vi "Test Suite Result Fail Count.vi"(8 "error in (no error)":errorcluster, 11 "Test Suite Result Test In":refnum<class "Test Suite Result Test.lvclass">) -> (0 "error out":errorcluster, 3 "Test Suite Result Test Out":refnum<class "Test Suite Result Test.lvclass">)   [LabVIEW 2020, in "LUnit Tests.lvlib" / "Test Suite Result Test.lvclass"]
uses:
  Test Suite Result Test.lvclass
  C:/Program Files (x86)/National Instruments/LabVIEW 2020/vi.lib/Asteme/LUnit/Test Case.lvclass
  source/Examples/Basic Example/Failing Test Case/Failing Test Case.lvclass
  C:/Users/anton/Documents/GitHub/LUnit/source/Framework/Test Case/LUnit Test Case.lvclass
  source/Framework/Result Classes/Test Suite Result/Test Suite Result.lvclass/Test Suite Result.ctl
  source/Framework/Result Classes/Test Case Result/Test Case Result.lvclass/Test Case Result.ctl
  source/Framework/Result Classes/Method Result/Method Result.lvclass/Method Result.ctl
  <vilib>/Asteme/LUnit/Test Case.lvclass/Test Case.ctl
  <vilib>/Asteme/LUnit/LUnit Assertion Result.lvclass/LUnit Assertion Result.ctl
  <vilib>/Asteme/LUnit/LUnit Test Case Result.lvclass/LUnit Test Case Result.ctl
  <vilib>/Asteme/LUnit/LUnit Method Result.lvclass/LUnit Method Result.ctl
  source/Framework/Result Classes/Test Suite Result/Private/SubVIs/Count by Status.vi
  <vilib>/Asteme/LUnit/Palette/Pass.vi
  <vilib>/Asteme/LUnit/Palette/Fail.vi
  <vilib>/Asteme/LUnit/Variant to string.vi
  <vilib>/Asteme/LUnit/Set Assertion Type.vi
  source/Framework/Result Classes/Test Case Result/Public/Accessors/Read Status.vi
  <vilib>/Asteme/LUnit/Add test result.vi
  <vilib>/Asteme/LUnit/LUnit Write Passed.vi
  <vilib>/Asteme/LUnit/LUnit Write Message.vi
  <vilib>/Asteme/LUnit/LUnit Write Description.vi
  <vilib>/Asteme/LUnit/LUnit Write Assertion Type.vi
  source/Framework/Result Classes/Test Case Result/Private/SubVIs/Merge Status.vi
  source/Framework/Result Classes/Method Result/Public/Read Status.vi
  <vilib>/Asteme/LUnit/LUnit Record Assertion Result.vi
  <vilib>/Asteme/LUnit/LUnit Aggregate Assertion Results.vi
  <vilib>/Asteme/LUnit/Assertion Result/LUnit Read Status.vi
  <vilib>/Asteme/LUnit/LUnit Read Message.vi
  <vilib>/Asteme/LUnit/LUnit Read Description.vi
  <vilib>/Asteme/LUnit/Method Result/LUnit Merge Status.vi
  <vilib>/Asteme/LUnit/LUnit Concatenate result strings.vi
  <vilib>/Utility/Data Type/Get Type Information.vi
  <vilib>/Utility/LVClass/Get LV Class Name.vi
  <vilib>/Asteme/LUnit/LUnit Assertion Result.lvclass
  <vilib>/Asteme/LUnit/Test Case.lvclass
  source/Framework/Result Classes/Test Suite Result/Test Suite Result.lvclass
  C:/Users/anton/Documents/GitHub/LUnit/source/Examples/Basic Example/Failing Test Case/Failing Test Case.lvclass
  C:/Users/anton/Documents/GitHub/LUnit/tests/Framework Test/Test Suite Result/Test Suite Result Test.lvclass
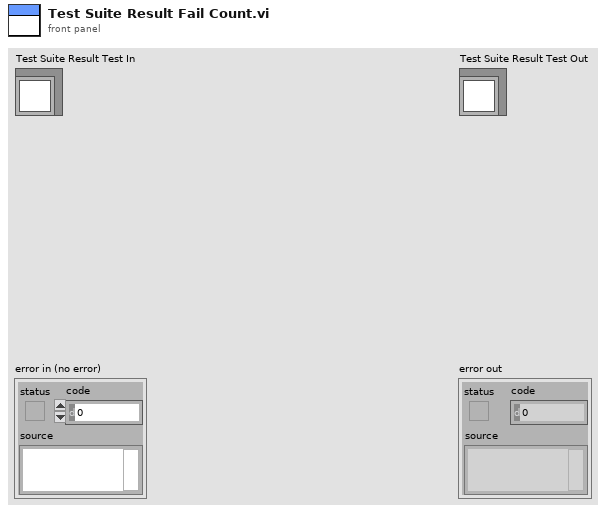
[diagram p1: front panel]
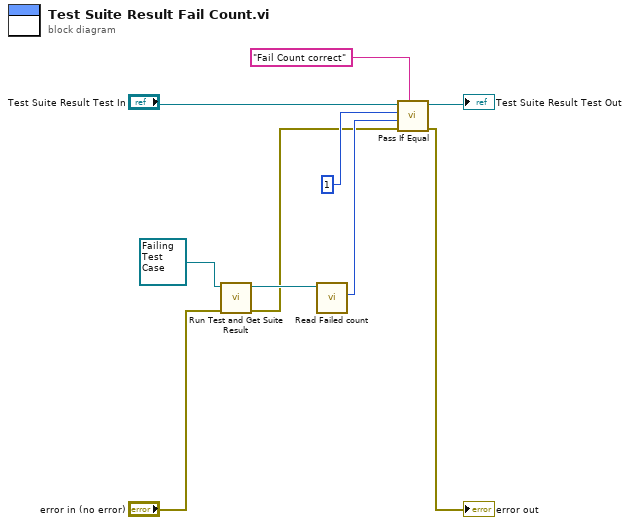
[diagram p0: block diagram]
diagram:
  n1 = call "Run Test and Get Suite Result.vi"("error in (no error)"="error in (no error)", "Test Test Case in"=refnum<class "Failing Test Case.lvclass"> refnum ("Failing Test Case.lvclass")) -> ("error out"=w3:errorcluster, "Test Suite Result out"=w4:refnum<class "Test Suite Result.lvclass">)  [unwired: 8 in]
  n2 = call "Read Failed count.vi"("Test Suite Result In"=w4) -> ("Failures count"=w9:i32)  [unwired: 8 in, 2 out]
  n3 = call <vilib>:"Pass If Equal.vi"("Description"="Fail Count correct", "error in (no error)"=w3, "Actual"=w9, "Expected"=1 ("x"), "LUnit Test Case In"="Test Suite Result Test In") -> ("error out"=→"error out":errorcluster, "LUnit Test Case Out"=→"Test Suite Result Test Out":refnum<class "Test Suite Result Test.lvclass">)  [unwired: 5 in]
